vi "rx_ed.vi"(8 "min_len":i32, 9 "Threshold":dbl=-40.0 format="%#_13g", 11 "Wavefrom":cluster{"t0":dbl, "dt":dbl, cdb[]}) -> (0 "avg energy":dbl, 3 "extract wav":cluster{"t0":dbl, "dt":dbl, cdb[]}[](array[cluster]))   [LabVIEW 2014]
uses:
  <vilib>/Analysis/baseanly.llb/Mean (DBL).vi
  <vilib>/Analysis/NI_AALBase.lvlib
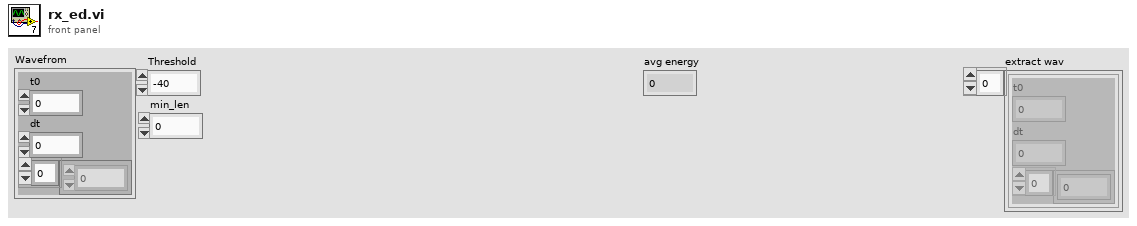
[diagram p1: front panel]
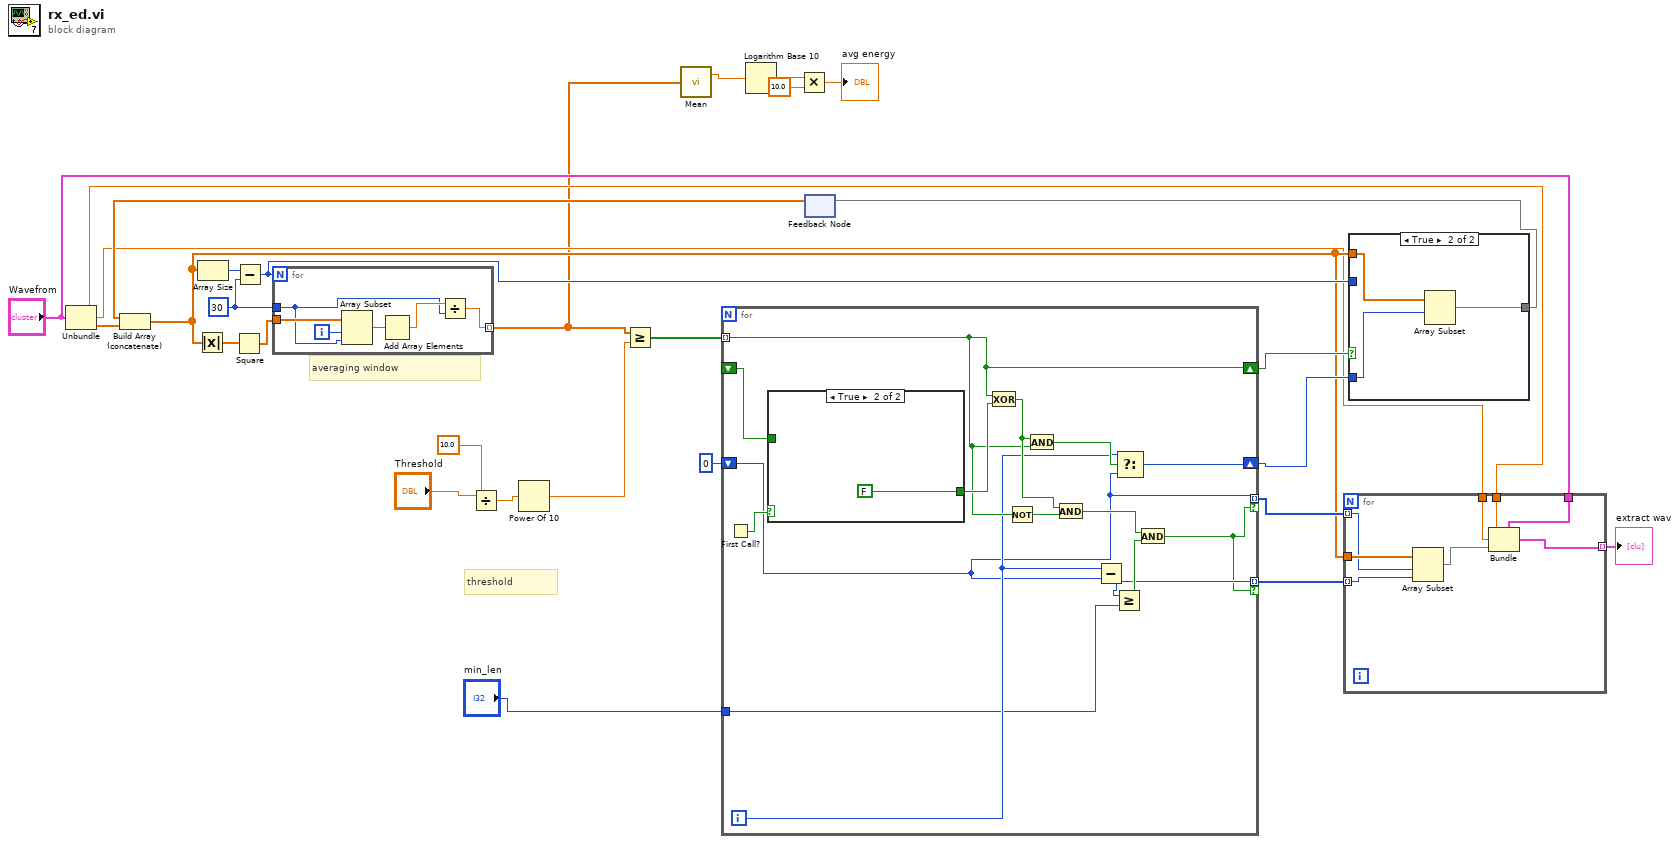
[diagram p0: block diagram]
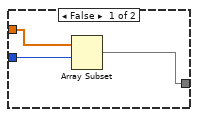
[diagram p2: hidden frame]
diagram:
  w27 = 30 ("y")
  # "averaging window"
  # "threshold"
  n1 = Unbundle("Wavefrom") -> ("t0"=w8:dbl, "dt"=w9:dbl, w16:cdb[])
  n2 = Divide(x="Threshold", y=10.0) -> (x/y=w23:dbl)
  n3 = Power Of 10(x=w23) -> (10^x=w22:dbl)
  n4 = feedback #1() -> (w14:cdb[])  [unwired: 1 in]
  n5 = Build Array (concatenate)(w14, w16) -> (w10:cdb[])
  n6 = Absolute Value(x=w10) -> (abs(x)=w28:dbl[])
  n7 = Array Size(array=w10) -> (size(s)=w29:i32)
  n8 = Square(x=w28) -> (x^2=w26:dbl[])
  n9 = Subtract(x=w29, y=w27) -> (x-y=w13:i32)
  n10 = for {
    N: w13 -> [_]
    tunnel: w26 -> [w35]
    tunnel: w27 -> [w31]
    tunnel: [w30] -> w5 mode=indexing
    i -> [w34]
    n11 = Array Subset(array=w35, index=w34, length=w31) -> (w33:dbl[])
    n12 = Add Array Elements(numeric array=w33) -> (sum=w32:dbl)
    n13 = Divide(x=w32, y=w31) -> (x/y=w30:dbl)
  }
  n14 = Greater Or Equal?(x=w5, y=w22) -> (x >= y?=w21:bool[])
  n15 = call-poly <vilib>:"Mean.vi"("X"=w5) -> ("mean"=w4:dbl)  [unwired: 1 out]
  n16 = for {
    tunnel: w21 -> [w44] mode=indexing
    shift-right: [w47] -> w17
    shift-left: 0 -> [w36]
    shift-right: [w44] -> w18
    shift-left: _ -> [w43]
    tunnel: "min_len" -> [w41]
    tunnel: [w36] -> w12 mode=indexing if=w37
    tunnel: [w38] -> w11 mode=indexing if=w37
    i -> [w42]
    n17 = First Call?() -> (First Call?: T/F=w50:bool)
    n18 = case shown="True" w50 {
      tunnel: [w51 FALSE] -> w49
      tunnel: w43 -> [w51 _]
      frame False {
      }
      frame True {
      }
    }
    n19 = Exclusive Or(1:w49, 2:w44) -> (0:w46:bool)
    n20 = Not(x=w44) -> (.not. x?=w45:bool)
    n21 = And(x=w46, y=w44) -> (x .and. y?=w48:bool)
    n22 = And(x=w46, y=w45) -> (x .and. y?=w40:bool)
    n23 = Subtract(x=w42, y=w36) -> (x-y=w38:i32)
    n24 = Greater Or Equal?(x=w38, y=w41) -> (x >= y?=w39:bool)
    n25 = Select(t=w42, s=w48, f=w36) -> (s? t:f=w47:i32)
    n26 = And(x=w40, y=w39) -> (x .and. y?=w37:bool)
  }
  n27 = Logarithm Base 10(1:w4) -> (0:w3:dbl)
  n28 = Multiply(x=w3, y=10.0) -> (x*y=→"avg energy":dbl)
  n29 = for {
    tunnel: w12 -> [w59] mode=indexing
    tunnel: w11 -> [w58] mode=indexing
    tunnel: w10 -> [w60]
    tunnel: w9 -> [w56]
    tunnel: w8 -> [w55]
    tunnel: "Wavefrom" -> [w54]
    tunnel: [w53] -> w6 mode=indexing
    n30 = Array Subset(array=w60, index=w59, length=w58) -> (w57:cdb[])
    n31 = Bundle(cluster=w54, "t0"=w55, "dt"=w56, w57) -> (w53:cluster{"t0":dbl, "dt":dbl, cdb[]})
  }
  "extract wav" <- w6
  n32 = case shown="True" w18 {
    tunnel: w17 -> [_ w66]
    tunnel: [w61 w65] -> w15
    tunnel: w10 -> [w63 w64]
    tunnel: w13 -> [w62 _]
    frame False {
      n33 = Array Subset(array=w63, index=w62) -> (w61:cdb[])  [unwired: 1 in]
    }
    frame True {
      n34 = Array Subset(array=w64, index=w66) -> (w65:cdb[])  [unwired: 1 in]
    }
  }
  n35 = feedback-in #1(w15) -> ()
